vi "Global Data.vi"() -> ()   [LabVIEW 2015, in "PL Model.lvlib"]
uses:
  PL Model.lvlib
panel:
  out "Main Loop Stop?":bool
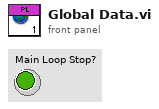
[diagram p1: front panel]
diagram:
